vi "onBoard button.vi"(8 "error in":errorcluster) -> (0 "error out":errorcluster, 10 "OnBoard.BUTTON":bool)   [LabVIEW 2019, in "my FPGA lib.lvlib"]
uses:
  my FPGA lib.lvlib
  <vilib>/Utility/error.llb/Error Cluster From Error Code.vi
  <vilib>/rvi/errors/niLvFpgaAdjustHostInterfaceError.vi
  <vilib>/rvi/interface/nirviReadWriteControl/nirviReadWriteControl.xnode
  NiFpgaLv.dll
  <vilib>/rvi/interface/Simulation/niFpgaSimulationCallBeginRW.vi
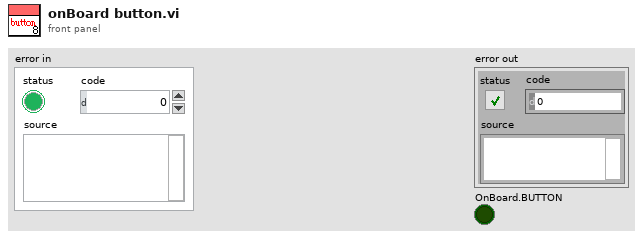
[diagram p1: front panel]
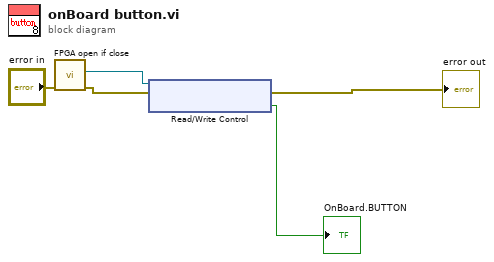
[diagram p0: block diagram]
diagram:
  n1 = call "FPGA open if close.vi"("error in"="error in") -> ("error out"=w3:errorcluster, "FPGA VI Reference Out"=w4:refnum<k20>)  [unwired: 9 in]
  n2 = xnode "Read/Write Control"("FPGA VI Reference In"=w4, "error in"=w3) -> ("error out"=→"error out":errorcluster, "OnBoard.BUTTON"=→"OnBoard.BUTTON":bool)  [unwired: 1 out]
